vi "get State.vi"(10 "state":i32, 11 "devID":u32) -> (2 "state out":i32, 3 "function return":i32)   [LabVIEW 2014, in "libchaos-driver-powersupply-labview.lvlib"]
doc: "int getState(unsigned int devID,int*state);"
uses:
  libchaos-driver-powersupply-labview.lvlib
  chaos-i686-dynamic-release/lib/libchaos-driver-powersupply-labview.so
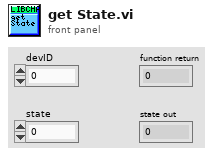
[diagram p1: front panel]
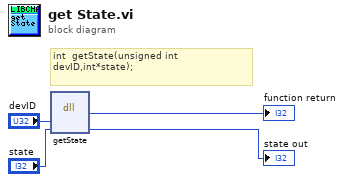
[diagram p0: block diagram]
diagram:
  # "int  getState(unsigned int devID,int*state);"
  n1 = dll-call lib="home/chaos/chaos_bundle/chaos-i686-dynamic-release/lib/libchaos-driver-powersupply-labview.*" fn="getState"("devID"="devID", "state"="state") -> (→"function return":i32, "state"=→"state out":i32)  [unwired: 4 in, 2 out]
